vi "Trajectory_selection.vi"(8 "Matrices":T1) -> (0 "test":dbl[][](array[numeric]))   [LabVIEW 2021]
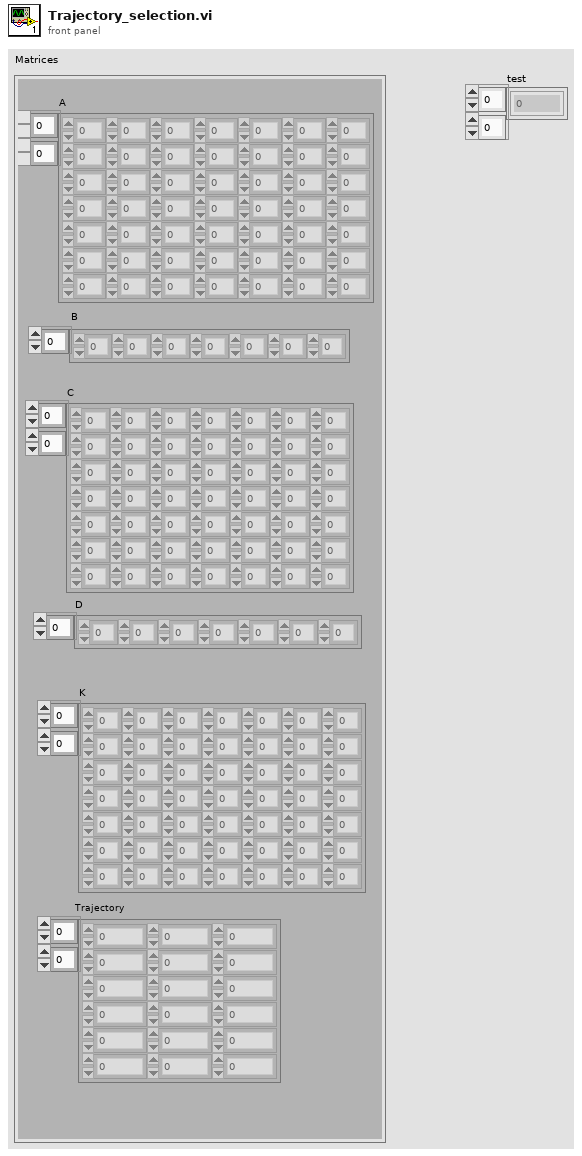
[diagram p1: front panel]
types:
  T1 = cluster{"B":dbl[], "A":dbl[][], "C":dbl[][], "D":dbl[], "K":dbl[][], "Trajectory":dbl[][]}
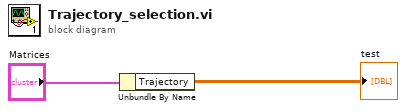
[diagram p0: block diagram]
diagram:
  n1 = Unbundle By Name("Matrices") -> ("Trajectory"=→"test":dbl[][])
